vi "example-tx-c_api.vi"() -> ()   [LabVIEW 2024]
uses:
  <vilib>/Analysis/1siggen.llb/Ramp Pattern by Samples.vi
  uhd (generated from wizard into user.lib - manually fixed for rx example)/uhd.lvlib
  <vilib>/Analysis/NI_AALBase.lvlib
  <vilib>/measure/NI_MABase.lvlib
panel:
  out "ant_out out":string
  in  "stop":bool
  out "freq_out out":dbl
  in  "target_freq":dbl=1000000000.0 format="%#_6p"
  in  "ant":string="TX/RX"
  out "gain_out out":dbl
  in  "gain":dbl
  out "rate_out out":dbl
  in  "rate":dbl=1000000.0 format="%#_6p"
  in  "chan":u64
  out "error out":errorcluster
  in  "args":string="type=b200"
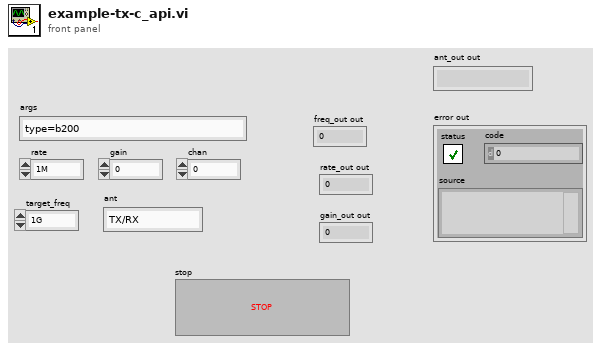
[diagram p1: front panel]
types:
  T1 = cluster{"cpu_format":string, "otw_format":string, "args":string, "channel_list":u64[], "n_channels":u64}
  T2 = cluster{"target_freq":dbl, "rf_freq_policy":u32, "@dummy control@":i8, "@dummy control@":i8, "@dummy control@":i8, "@dummy control@":i8, "rf_freq":dbl, "dsp_freq_policy":u32, "@dummy control@":i8, "@dummy control@":i8, "@dummy control@":i8, "@dummy control@":i8, "dsp_freq":dbl, "args":u64}
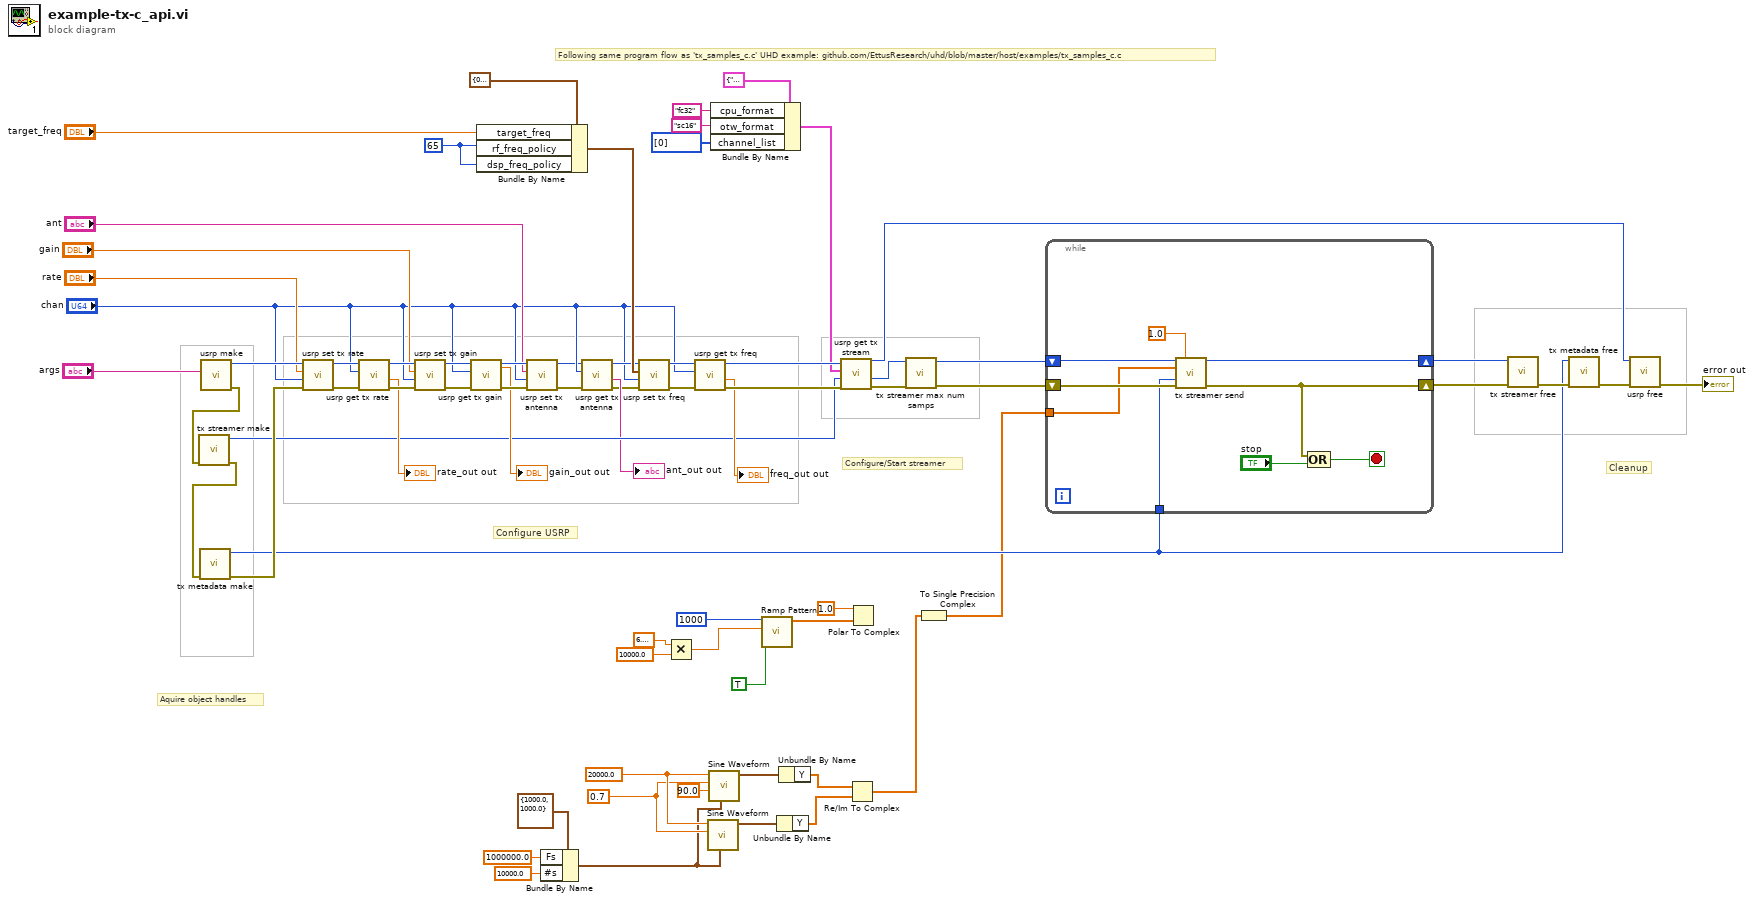
[diagram p0: block diagram]
diagram:
  w11 = 0.7 ("amplitude")
  w12 = 20000.0 ("frequency")
  w29 = u32 65 ("rf_freq_policy")
  # "Cleanup"
  # "Configure/Start streamer"
  # "Configure USRP"
  # "Aquire object handles"
  # "Following same program flow as 'tx_samples_c.c' UHD example: github.com/EttusResearch/uhd/blob/master/host/examples/tx_samples_c.c"
  n1 = call "usrp make.vi"("args"="args") -> ("error out"=w70:errorcluster, "h"=w68:u64)  [unwired: 8 in, 1 out]
  n2 = call "tx streamer make.vi"("error in (no error)"=w70) -> ("error out"=w54:errorcluster, "h out"=w26:u64)  [unwired: 8 in, 1 out]
  n3 = call "tx metadata make.vi"("error in (no error)"=w54) -> ("error out"=w67:errorcluster, "handle out"=w20:u64)  [unwired: 8 in, 1 out]
  n4 = call "usrp set tx rate.vi"("error in (no error)"=w67, "chan"="chan", "rate"="rate", "h"=w68) -> ("error out"=w66:errorcluster, "h 2"=w53:u64)  [unwired: 5 in, 1 out]
  n5 = call "usrp get tx rate.vi"("error in (no error)"=w66, "chan"="chan", "h"=w53) -> ("error out"=w65:errorcluster, "rate_out out"=→"rate_out out":dbl, "h 2"=w52:u64)  [unwired: 5 in, 1 out]
  n6 = call "usrp set tx gain.vi"("error in (no error)"=w65, "chan"="chan", "gain"="gain", "h"=w52) -> ("error out"=w64:errorcluster, "h 2"=w51:u64)  [unwired: 5 in, 1 out]
  n7 = call "usrp get tx gain.vi"("error in (no error)"=w64, "chan"="chan", "h"=w51) -> ("error out"=w63:errorcluster, "h 2"=w50:u64, "gain_out out"=→"gain_out out":dbl)  [unwired: 5 in, 1 out]
  n8 = Bundle By Name(cluster=T2 {"target_freq"=0.0, "rf_freq_policy"=78, "@dummy control@"=0, "@dummy control@"=0, "@dummy control@"=0, "@dummy control@"=0, "rf_freq"=0.0, "dsp_freq_policy"=78, "@dummy control@"=0, "@dummy control@"=0, "@dummy control@"=0, "@dummy control@"=0, "dsp_freq"=0.0, "args"=0} ("tune_request"), "target_freq"="target_freq", "rf_freq_policy"=w29, "dsp_freq_policy"=w29) -> (w28:T2)
  n9 = call "usrp set tx antenna.vi"("error in (no error)"=w63, "chan"="chan", "ant"="ant", "h"=w50) -> ("error out"=w16:errorcluster, "h 2"=w17:u64)  [unwired: 5 in, 1 out]
  n10 = Bundle By Name(cluster=cluster{"Fs":dbl, "#s":dbl} {"Fs"=1000.0, "#s"=1000.0} ("sampling info"), "Fs"=1000000.0, "#s"=10000.0) -> (w6:cluster{"Fs":dbl, "#s":dbl})
  n11 = call "usrp get tx antenna.vi"("error in (no error)"=w16, "chan"="chan", "h"=w17) -> ("error out"=w14:errorcluster, "ant_out out"=→"ant_out out":string, "h 2"=w19:u64)  [unwired: 5 in, 1 out]
  n12 = call "usrp set tx freq.vi"("error in (no error)"=w14, "chan"="chan", "tune_request"=w28, "h"=w19) -> ("error out"=w62:errorcluster, "h 2"=w49:u64)  [unwired: 2 in, 4 out]
  n13 = Multiply(x=6.283185307179586, y=10000.0) -> (x*y=w39:dbl)
  n14 = call "usrp get tx freq.vi"("error in (no error)"=w62, "chan"="chan", "h"=w49) -> ("error out"=w61:errorcluster, "freq_out out"=→"freq_out out":dbl, "h 2"=w48:u64)  [unwired: 5 in, 1 out]
  n15 = call <vilib>:"Sine Waveform.vi"("sampling info"=w6, "amplitude"=w11, "frequency"=w12) -> ("signal out"=w4:waveform(dbl))  [unwired: 7 in, 1 out]
  n16 = call <vilib>:"Sine Waveform.vi"("sampling info"=w6, "phase"=90.0, "amplitude"=w11, "frequency"=w12) -> ("signal out"=w5:waveform(dbl))  [unwired: 6 in, 1 out]
  n17 = Bundle By Name(cluster=T1 {"cpu_format"="", "otw_format"="", "args"="", "channel_list"=[], "n_channels"=0} ("stream_args 2"), "cpu_format"="fc32", "otw_format"="sc16", "channel_list"=u64[] [0]) -> (w21:T1)
  n18 = call-poly <vilib>:"Ramp Pattern.vi"("exclude end?"=TRUE, "end"=w39, "samples"=1000) -> ("Ramp Pattern"=w43:dbl[])  [unwired: 7 in, 1 out]
  n19 = Unbundle By Name(w4) -> ("Y"=w2:dbl[])
  n20 = Unbundle By Name(w5) -> ("Y"=w3:dbl[])
  n21 = call "usrp get tx stream.vi"("error in (no error)"=w61, "h_out"=w26, "stream_args 2"=w21, "h"=w48) -> ("error out"=w60:errorcluster, "h_out 2"=w47:u64, "h 2"=w46:u64)  [unwired: 3 in, 2 out]
  n22 = Re/Im To Complex(1:w2, 2:w3) -> (0:w1:cdb[])
  n23 = Polar To Complex(1:w43, 2:1.0 ("r")) -> ()  [unwired: 1 out]
  n24 = call "tx streamer max num samps.vi"("error in (no error)"=w60, "h"=w47) -> ("error out"=w59:errorcluster, "h 2"=w45:u64)  [unwired: 6 in, 2 out]
  n25 = To Single Precision Complex(1:w1) -> (0:w13:csg[])
  n26 = while {
    shift-right: [w77] -> w44
    shift-left: w45 -> [w78]
    shift-right: [w72] -> w56
    shift-left: w59 -> [w79]
    tunnel: w13 -> [w76]
    tunnel: w20 -> [w74]
    stop <- w71 stop-if-true
    n27 = call "tx streamer send.vi"("h"=w78, "timeout"=1.0, "buffs"=w76, "md"=w74, "error in (no error)"=w79) -> ("h 2"=w77:u64, "error out"=w72:errorcluster)  [unwired: 5 in, 4 out]
    n28 = Compound Arithmetic op=OR(w72, "stop") -> (w71:bool)
  }
  n29 = call "tx streamer free.vi"("error in (no error)"=w56, "h"=w44) -> ("error out"=w57:errorcluster)  [unwired: 7 in, 2 out]
  n30 = call "tx metadata free.vi"("error in (no error)"=w57, "handle"=w20) -> ("error out"=w58:errorcluster)  [unwired: 7 in, 2 out]
  n31 = call "usrp free.vi"("error in (no error)"=w58, "h"=w46) -> ("error out"=→"error out":errorcluster)  [unwired: 7 in, 2 out]
